vi "Build Data Log Path.vi"(8 "error in (no error)":errorcluster) -> (0 "error out":errorcluster, 3 "appended path":path)   [LabVIEW 2026, in "Data Logging.lvlib"]
uses:
  Data Logging.lvlib
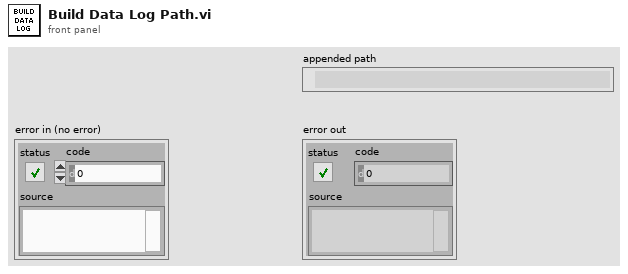
[diagram p1: front panel]
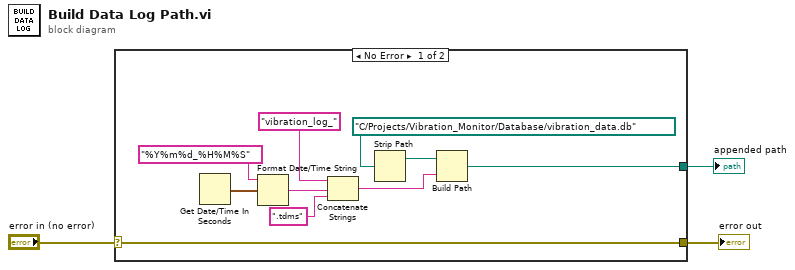
[diagram p0: block diagram]
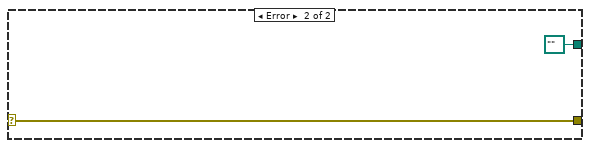
[diagram p2: hidden frame]
diagram:
  n1 = case shown="No Error" "error in (no error)" {
    selector: "error in (no error)" -> [w4 w15]
    tunnel: [w6 path "" ("appended path")] -> w3
    tunnel: [w4 w15] -> w1
    frame No Error {
      n2 = Get Date/Time In Seconds() -> (seconds since 1Jan1904=w7:timestamp)
      n3 = Format Date/Time String(time format string (%c)="%Y%m%d_%H%M%S" ("format string"), seconds (now)=w7) -> (date/time string=w8:string)  [unwired: 1 in]
      n4 = Concatenate Strings("vibration_log_" ("format string"), w8, ".tdms" ("format string")) -> (w12:string)
      n5 = Strip Path(path=path "C:/Projects/Vibration_Monitor/Database/vibration_data.db") -> (stripped path=w5:path)  [unwired: 1 out]
      n6 = Build Path(base path=w5, name or relative path=w12) -> (appended path=w6:path)
    }
    frame Error {
    }
  }
  "appended path" <- w3
  "error out" <- w1
